vi "CODMn通讯.vi"() -> ()   [LabVIEW 2016, in "斯坦道CODMn新电路板.lvlib"]
uses:
  <vilib>/NI/Modbus Library/API/Wrapper/Create TCP Slave.vi
  <vilib>/Utility/config.llb/Write Key (String).vi
  <vilib>/Plasmionique/MB Master/MB_Master/MB_Master.lvclass
  <vilib>/NI/Modbus Library/API/slave/Modbus Slave.lvclass
  <vilib>/Utility/config.llb/NI_LVConfig.lvlib
  <vilib>/Plasmionique/MB Master/MB Master.lvlib
  <vilib>/NI/Modbus Library/API/Wrapper/API Main.lvlib
panel:
  out "控制命令 2":u16[](array[numeric]) format="%xH"
  out "状态告警区":T1 {"工作状态" items=["空闲"=0, "水样测试"=1, "标样核查"=2, "零点核查"=3, "跨度核查"=4, "空白测试"=5, "平行样测试"=6, "加标回收"=7, "空白校准"=8, "标样校准"=9, "初始化（清洗）"=10, "调试"=22, "填充管路"=30, "清洗管路"=31, "清洗反应杯"=32]; "告警代码" items=["无告警", "缺试剂告警", "缺水样告警", "缺蒸馏水告警", "缺标液告警", "仪表漏液告警", "标定异常告警", "超量程告警", "加热异常", "低试剂预警", "超上限告警", "超下限告警", "仪表内部其他异常", "滴定异常告警", "电极异常告警", "量程切换告警", "参数设置告警", "PH电极电位异常", "电导率电极异常", "浊度光度异常", "溶解氧电极异常", "溶解氧光强异常", "温度异常告警", "PH异常告警", "溶解氧异常告警", "电导率异常告警", "浊度异常告警", "叶绿素异常告警", "藻密度异常告警", "蓝绿藻异常告警", "ORP异常告警", "氨氮异常告警", "清洁刷异常告警", "SD卡异常告警", "蓝牙异常告警", "Wifi异常告警", "流程异常告警"]; "故障代码" items=["无故障", "电机故障", "温度故障", "通讯故障", "滴定故障"]}
  out "测量数据区":T2 {"单位" items=["ug/L", "mg/L", "ppm", "mg/m3", "cm", "ppb", "ug/m3", "%", "nmol/mol", "umol/mol", "MPN/L", "MPN/100ml", "ng/m3", "NTU", "无量纲", "ms/cm", "us/cm", "℃", "mV", "万个/L"]}
  out "状态告警区":u16[](array[numeric])
  out "测量数据区":u16[](array[numeric])
  out "序列号":string
  out "status":bool
  out "关键参数区":T3
  in  "读关键参数区":bool
  in  "读状态告警区":bool
  in  "读测量数据区":bool
  in  "站号":u16(ring) items=["CODMn"=21, "氨氮"=3]
  in  "停止":bool
  in  "启动":bool
  in  "控制命令":u16(ring) items=["启动测量"=1, "标样核查"=2, "零点核查"=3, "跨度核查"=4, "空白测试"=5, "平行样测试"=6, "加标回收"=7, "空白校准"=8, "标样校准"=9, "初始化（清洗）"=10, "停止测试"=11, "仪器重启"=12, "校时"=13, "模式设置"=14, "测量间隔设置"=15]
  in  "控制命令参数":u16[](array[numeric]) format="%04xH"
  in  "VISA Resource":refnum<visa-resource-name>
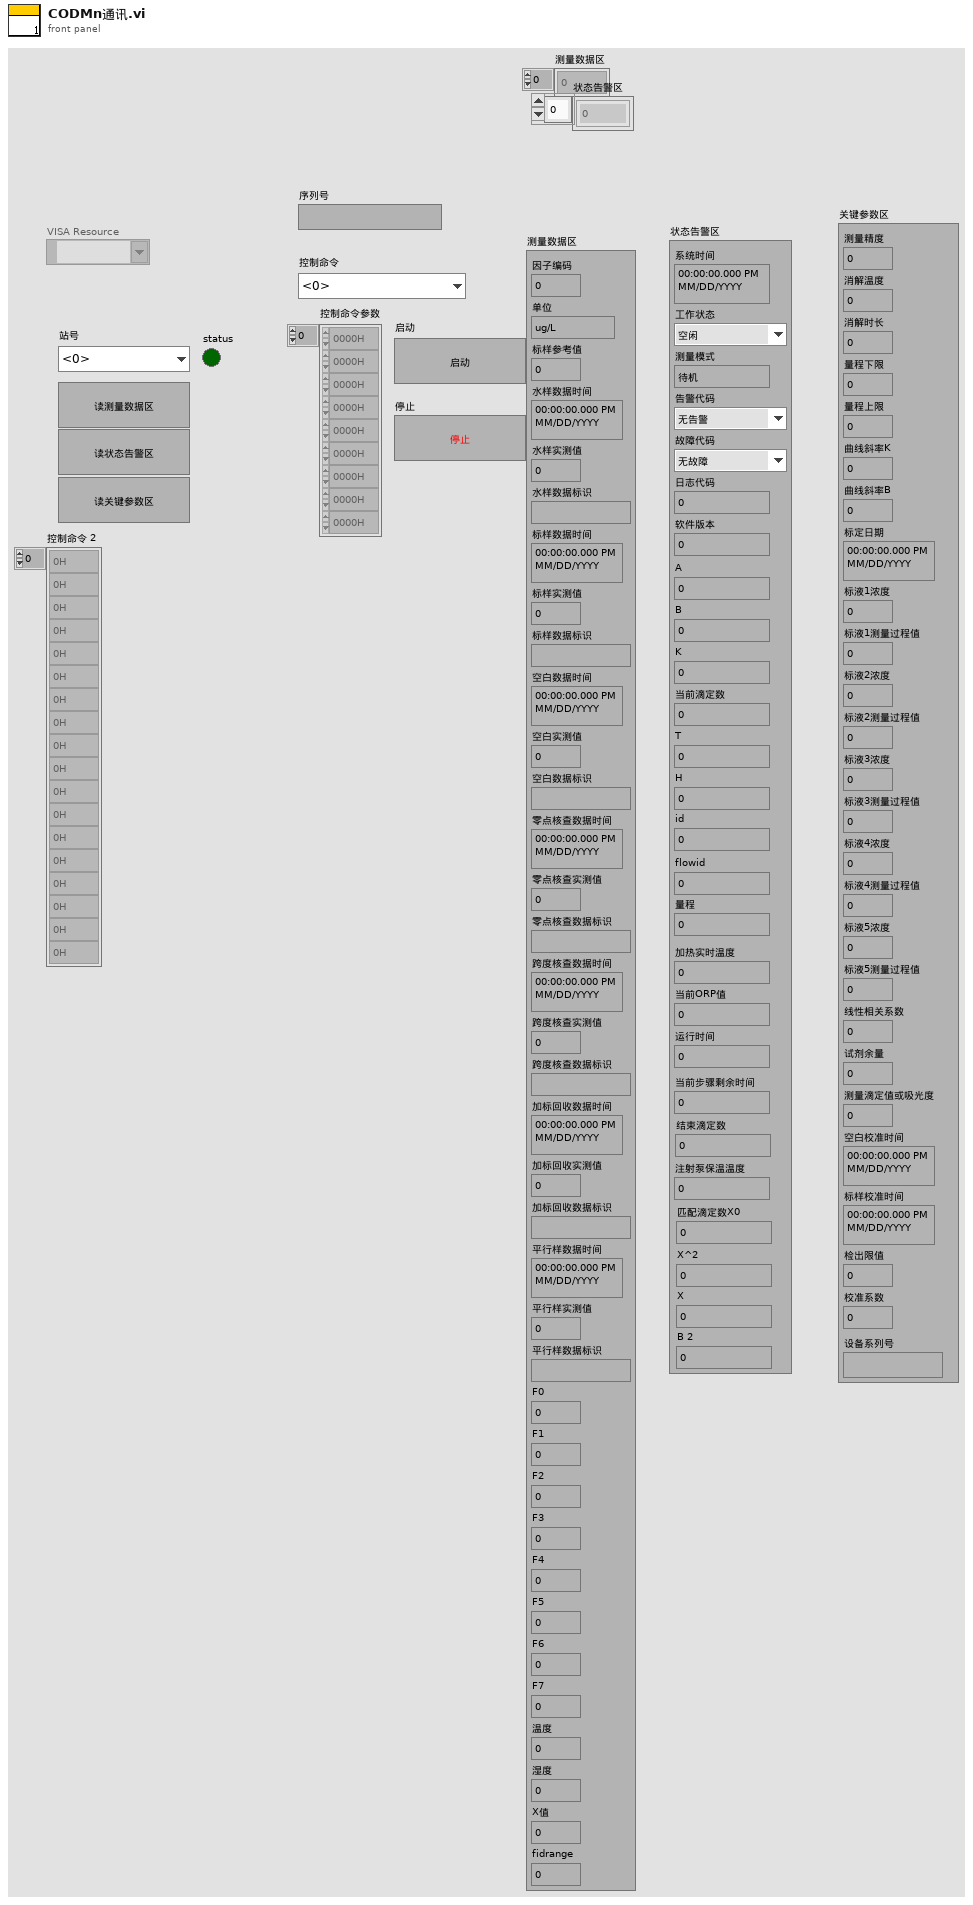
[diagram p1: front panel]
types:
  T1 = cluster{"系统时间":timestamp, "工作状态":u16, "测量模式":enum16{"待机", "连续模式", "周期模式", "定点模式", "受控模式", "手动模式"}, "告警代码":u16, "故障代码":u16, "日志代码":u16, "软件版本":u16, "A":sgl, "B":sgl, "K":sgl, "当前滴定数":sgl, "T":sgl, "H":sgl, "id":u16, "flowid":u16, "量程":u16, "加热实时温度":sgl, "当前ORP值":sgl, "运行时间":sgl, "当前步骤剩余时间":sgl, "结束滴定数":sgl, "注射泵保温温度":sgl, "匹配滴定数X0":u16, "X^2":sgl, "X":sgl, "B 2":sgl}
  T2 = cluster{"因子编码":u32, "单位":u16, "标样参考值":sgl, "水样数据时间":timestamp, "水样实测值":sgl, "水样数据标识":string, "标样数据时间":timestamp, "标样实测值":sgl, "标样数据标识":string, "空白数据时间":timestamp, "空白实测值":sgl, "空白数据标识":string, "零点核查数据时间":timestamp, "零点核查实测值":sgl, "零点核查数据标识":string, "跨度核查数据时间":timestamp, "跨度核查实测值":sgl, "跨度核查数据标识":string, "加标回收数据时间":timestamp, "加标回收实测值":sgl, "加标回收数据标识":string, "平行样数据时间":timestamp, "平行样实测值":sgl, "平行样数据标识":string, "F0":sgl, "F1":sgl, "F2":sgl, "F3":sgl, "F4":sgl, "F5":sgl, "F6":sgl, "F7":sgl, "温度":sgl, "湿度":sgl, "X值":sgl, "fidrange":sgl}
  T3 = cluster{"测量精度":u16, "消解温度":u16, "消解时长":u16, "量程下限":sgl, "量程上限":sgl, "曲线斜率K":sgl, "曲线斜率B":sgl, "标定日期":timestamp, "标液1浓度":sgl, "标液1测量过程值":sgl, "标液2浓度":sgl, "标液2测量过程值":sgl, "标液3浓度":sgl, "标液3测量过程值":sgl, "标液4浓度":sgl, "标液4测量过程值":sgl, "标液5浓度":sgl, "标液5测量过程值":sgl, "线性相关系数":sgl, "试剂余量":u32, "测量滴定值或吸光度":sgl, "空白校准时间":timestamp, "标样校准时间":timestamp, "检出限值":sgl, "校准系数":sgl, "设备系列号":string}
  T4 = typedef "CODMn交互.ctl" = cluster{"COD浓度（mg/L)":dbl, "水样启动时间":timestamp, "加标回收启动时间":timestamp, "CODMn工作状态":enum16{"空闲", "水样测试", "标样核查", "零点核查", "跨度核查", "空白测试", "平行样测试", "加标回收", "空白校准", "标样校准", "初始化（清洗）"}, "多列列表框":i32, "平台试剂余量百分比":sgl, "CODMn仪器参数":cluster{"测量量程":dbl, "测量精度":dbl, "测量间隔":dbl, "消解温度":dbl, "消解时长":dbl, "空白校准时间":timestamp, "曲线截距":dbl, "曲线斜率":dbl, "测量检出限":dbl, "测量信号值":dbl, "线性相关系数":dbl, "二次多项式系数":dbl, "标样校准时间":timestamp, "稀释倍数":dbl, "三项式系数":dbl, "空白标定系数":dbl, "量程系数":dbl, "F0/ORPA":dbl, "F1/ORPB":dbl, "F2/ORPK":dbl, "F3":dbl, "F4":dbl, "F5":dbl, "F6":dbl, "F7":dbl, "X0/滴定数":dbl, "量程":dbl}}
  T5 = cluster{"测量模式":enum16{"水样测量", "标样核查", "零点核查", "跨度核查", "空白测试", "加标回收", "平行样", "校零", "校标"}}
  T6 = typedef "量程选择控件.ctl" = enum32{"L", "H", "AUTO"}
  T7 = cluster{"水样测试量程模式":T6, "标样核查量程模式":T6, "零点核查量程模式":T6, "跨度核查量程模式":T6, "空白测试量程模式":T6, "平行样测试量程模式":T6, "加标回收量程模式":T6, "空白校准量程模式":T6, "标样校准量程模式":T6}
  T8 = cluster{"测量量程":dbl, "测量精度":dbl, "测量间隔":dbl, "消解温度":dbl, "消解时长":dbl, "空白校准时间":timestamp, "曲线截距":dbl, "曲线斜率":dbl, "测量检出限":dbl, "测量信号值":dbl, "线性相关系数":dbl, "二次多项式系数":dbl, "标样校准时间":timestamp, "稀释倍数":dbl, "三项式系数":dbl, "空白标定系数":dbl, "量程系数":dbl, "F0/ORPA":dbl, "F1/ORPB":dbl, "F2/ORPK":dbl, "F3":dbl, "F4":dbl, "F5":dbl, "F6":dbl, "F7":dbl, "X0/滴定数":dbl, "量程":dbl}
  T9 = typedef "NI_LVConfig.lvlib/Config Data RefNum.ctl" = refnum<k1>
  T10 = cluster{"站号":u16, "量程切换":enum32{"H", "L", "AUTO"}, "控制命令":u16, "模式设置":enum16{"待机", "连续模式", "周期模式", "定点模式", "受控模式", "手动模式"}, "测量间隔":u16}
  T11 = enum16{"水样测量", "标样核查", "零点核查", "跨度核查", "空白测试", "加标回收", "平行样", "校零", "校标"}
  T12 = enum8{"Enabled", "Disabled", "Disabled and Grayed Out"}
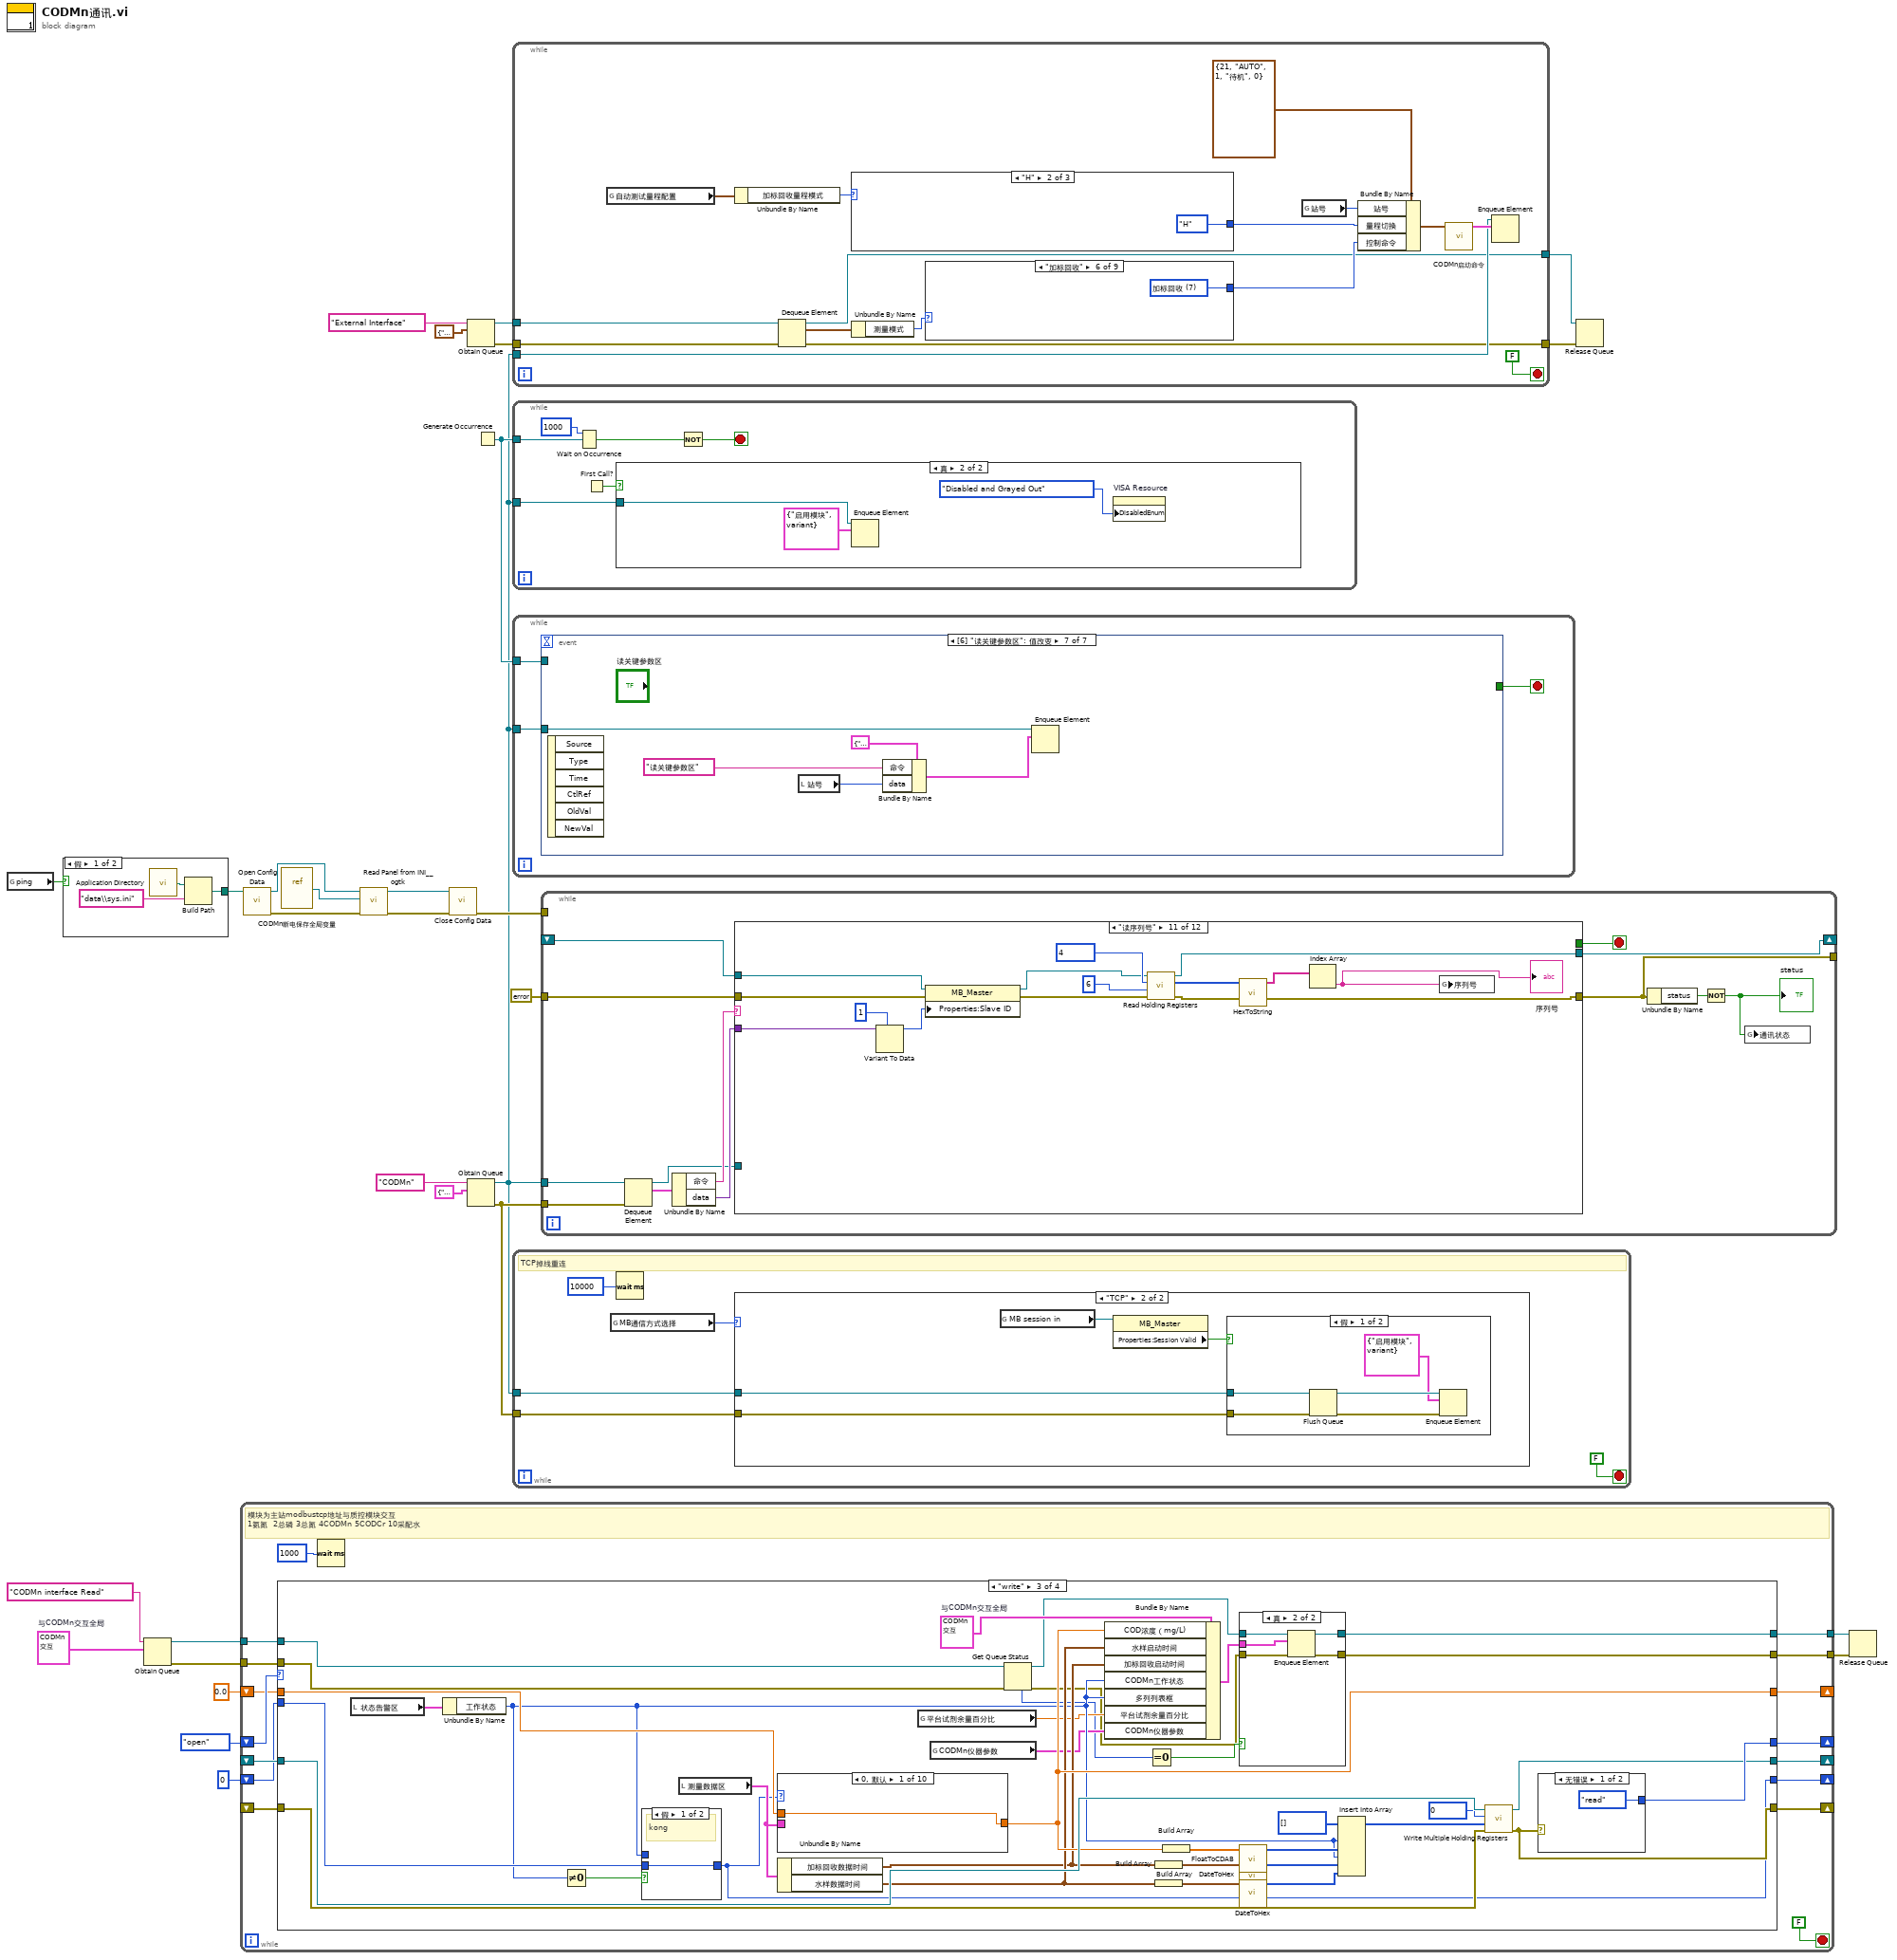
[diagram p0: block diagram]
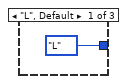
[diagram p2: hidden frame]
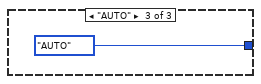
[diagram p3: hidden frame]
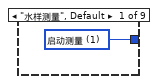
[diagram p4: hidden frame]
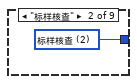
[diagram p5: hidden frame]
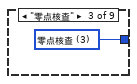
[diagram p6: hidden frame]
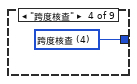
[diagram p7: hidden frame]
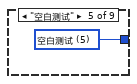
[diagram p8: hidden frame]
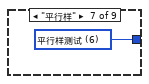
[diagram p9: hidden frame]
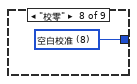
[diagram p10: hidden frame]
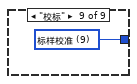
[diagram p11: hidden frame]
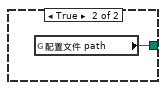
[diagram p12: hidden frame]
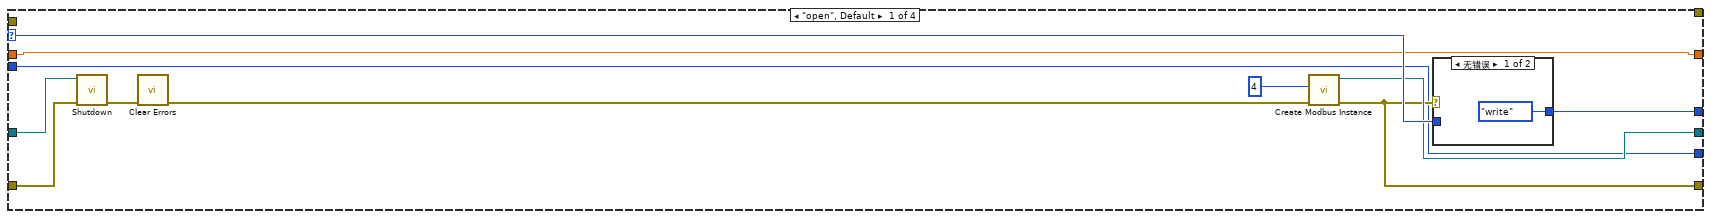
[diagram p15: hidden frame]
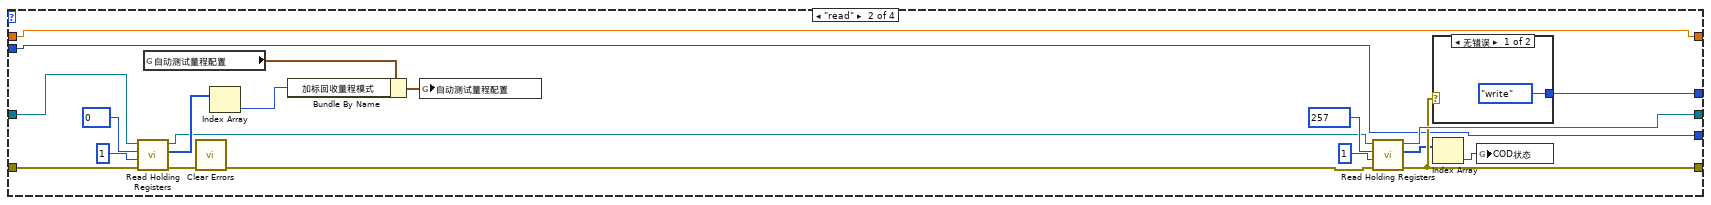
[diagram p17: hidden frame]
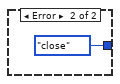
[diagram p18: hidden frame]
diagram:
  w4 = T4 {"COD浓度（mg/L)"=0.0, "水样启动时间"=timestamp(0 s since 1904-01-01), "加标回收启动时间"=timestamp(0 s since 1904-01-01), "CODMn工作状态"=enum."空闲", "多列列表框"=0, "平台试剂余量百分比"=0.0, "CODMn仪器参数"={"测量量程"=0.0, "测量精度"=0.0, "测量间隔"=0.0, "消解温度"=0.0, "消解时长"=0.0, "空白校准时间"=timestamp(0 s since 1904-01-01), "曲线截距"=0.0, "曲线斜率"=0.0, "测量检出限"=0.0, "测量信号值"=0.0, "线性相关系数"=0.0, "二次多项式系数"=0.0, "标样校准时间"=timestamp(0 s since 1904-01-01), "稀释倍数"=0.0, "三项式系数"=0.0, "空白标定系数"=0.0, "量程系数"=0.0, "F0/ORPA"=0.0, "F1/ORPB"=0.0, "F2/ORPK"=0.0, "F3"=0.0, "F4"=0.0, "F5"=0.0, "F6"=0.0, "F7"=0.0, "X0/滴定数"=0.0, "量程"=0.0}}  # 与CODMn交互全局
  n1 = global read "VARCODMn全局变量.vi" "ping"() -> (w17:bool)
  n2 = case shown="假" w17 {
    tunnel: [w30 w33] -> w16
    frame False {
      n3 = call <vilib>:"Application Directory.vi"() -> ("Application Directory"=w32:path)
      n4 = Build Path(base path=w32, name or relative path="data\\sys.ini" ("名称或相对路径")) -> (appended path=w30:path)
    }
    frame True {
      n5 = global read "VARCODMn全局变量.vi" "配置文件 path"() -> (w33:path)
    }
  }
  n6 = Obtain Queue(name (unnamed)="CODMn interface Read" ("写入方名称"), element data type=w4) -> (queue out=w6:refnum<queue>, error out=w1:errorcluster)  [unwired: 3 in, 1 out]
  n7 = while {
    shift-right: [w47] -> _
    shift-left: _ -> [w49]
    shift-right: [w46] -> _
    shift-left: _ -> [w48]
    shift-right: [w43] -> _
    shift-left: enum16{"open", "read", "write", "close"}."open" -> [w44]
    shift-right: [w41] -> _
    shift-left: sgl 0.0 ("标样实测值") -> [w40]
    shift-right: [w39] -> _
    shift-left: u16 0 ("工作状态") -> [w38]
    tunnel: w6 -> [w37]
    tunnel: [w36] -> w3
    tunnel: [w35] -> w2
    tunnel: w1 -> [w34]
    stop <- FALSE stop-if-true
    # "模块为主站modbustcp地址与质控模块交互\n1氨氮  2总磷 3总氮 4CODMn 5CODCr 10采配水"
    n8 = case shown="\"write\"" w44 {
      selector: w44 -> [w60 _ _ _]
      tunnel: w49 -> [w54 w70 w119 w155]
      tunnel: w48 -> [w53 w69 w118 w154]
      tunnel: [w57 w81 w116 w155] -> w47
      tunnel: [w56 w80 w115 w157] -> w46
      tunnel: [w59 w82 w120 enum16{"open", "read", "write", "close"}."open"] -> w43
      tunnel: [w51 w75 w99 w152] -> w41
      tunnel: w40 -> [w51 w75 w112 w152]
      tunnel: [w50 w74 w103 w151] -> w39
      tunnel: w38 -> [w50 w74 w102 w151]
      tunnel: w37 -> [_ _ w93 _]
      tunnel: [_ _ w91 _] -> w36
      tunnel: [_ _ w90 _] -> w35
      tunnel: w34 -> [_ _ w86 _]
      frame "open", Default {
        n9 = call-dynamic "Shutdown.vi"("error in"=w53, "Modbus slave in"=w54) -> ("error out"=w52:errorcluster)  [unwired: 9 in]
        n10 = call <vilib>:"Clear Errors.vi"("error in (no error)"=w52) -> ("error out"=w55:errorcluster)  [unwired: 5 in, 1 out]
        n11 = call-poly <vilib>:"Create Modbus Instance.vi"("error in"=w55, "port (502)"=u16 4) -> ("error out"=w56:errorcluster, "TCP slave instance"=w57:refnum<class "Modbus Slave.lvclass">)  [unwired: 8 in]
        n12 = case shown="无错误" w56 {
          tunnel: w60 -> [_ w62]
          tunnel: [enum16{"open", "read", "write", "close"}."write" w62] -> w59
          frame No Error {
          }
          frame Error {
          }
        }
      }
      frame "read" {
        n13 = call-dynamic <vilib>:"Read Holding Registers.vi"("error in"=w69, "number of inputs"=u16 1, "starting address"=u16 0, "Modbus slave in"=w70) -> ("error out"=w68:errorcluster, "register values"=w73:u16[], "Modbus slave out"=w67:refnum<class "Modbus Slave.lvclass">)  [unwired: 5 in]
        n14 = global read "CODMn断电保存全局变量.vi" "自动测试量程配置"() -> (w65:T7)
        n15 = call <vilib>:"Clear Errors.vi"("error in (no error)"=w68) -> ("error out"=w63:errorcluster)  [unwired: 5 in, 1 out]
        n16 = Index Array(array=w73) -> (element=w64:u16)  [unwired: 1 in]
        n17 = Bundle By Name(cluster=w65, "加标回收量程模式"=w64) -> (w66:T7)
        n18 = global write "CODMn断电保存全局变量.vi" "自动测试量程配置"(w66) -> ()
        n19 = call-dynamic <vilib>:"Read Holding Registers.vi"("error in"=w63, "number of inputs"=u16 1, "starting address"=u16 257, "Modbus slave in"=w67) -> ("error out"=w80:errorcluster, "register values"=w77:u16[], "Modbus slave out"=w81:refnum<class "Modbus Slave.lvclass">)  [unwired: 5 in]
        n20 = case shown="无错误" w80 {
          tunnel: [enum16{"open", "read", "write", "close"}."write" enum16{"open", "read", "write", "close"}."close"] -> w82
          frame No Error {
          }
          frame Error {
          }
        }
        n21 = Index Array(array=w77) -> (element=w76:u16)  [unwired: 1 in]
        n22 = global write "VARCODMn全局变量.vi" "COD状态"(w76) -> ()
      }
      frame "write" {
        w100 = T4 {"COD浓度（mg/L)"=0.0, "水样启动时间"=timestamp(0 s since 1904-01-01), "加标回收启动时间"=timestamp(0 s since 1904-01-01), "CODMn工作状态"=enum."空闲", "多列列表框"=0, "平台试剂余量百分比"=0.0, "CODMn仪器参数"={"测量量程"=0.0, "测量精度"=0.0, "测量间隔"=0.0, "消解温度"=0.0, "消解时长"=0.0, "空白校准时间"=timestamp(0 s since 1904-01-01), "曲线截距"=0.0, "曲线斜率"=0.0, "测量检出限"=0.0, "测量信号值"=0.0, "线性相关系数"=0.0, "二次多项式系数"=0.0, "标样校准时间"=timestamp(0 s since 1904-01-01), "稀释倍数"=0.0, "三项式系数"=0.0, "空白标定系数"=0.0, "量程系数"=0.0, "F0/ORPA"=0.0, "F1/ORPB"=0.0, "F2/ORPK"=0.0, "F3"=0.0, "F4"=0.0, "F5"=0.0, "F6"=0.0, "F7"=0.0, "X0/滴定数"=0.0, "量程"=0.0}}  # 与CODMn交互全局
        n23 = local read "状态告警区"() -> (w101:T1)
        n24 = Unbundle By Name(w101) -> ("工作状态"=w96:u16)
        n25 = Not Equal To 0?(x=w96) -> (x != 0?=w104:bool)
        n26 = case shown="假" w104 {
          tunnel: w96 -> [_ w129]
          tunnel: [w128 w129] -> w103
          tunnel: w102 -> [w128 _]
          frame False {
            # "kong"
          }
          frame True {
            # "..."
          }
        }
        n27 = local read "测量数据区"() -> (w109:T2)
        n28 = case shown="0, 默认" w103 {
          tunnel: [w130 w132 w134 w136 w138 w140 w142 w144 w146 w148] -> w99
          tunnel: w112 -> [w130 _ _ _ _ _ _ _ _ _]
          tunnel: w109 -> [_ w131 w133 w135 w137 w139 w141 w143 w145 w147]
          frame 0, Default {
          }
          frame 1 {
            n29 = Unbundle By Name(w131) -> ("水样实测值"=w132:sgl)
          }
          frame 2 {
            n30 = Unbundle By Name(w133) -> ("标样实测值"=w134:sgl)
          }
          frame 3 {
            n31 = Unbundle By Name(w135) -> ("零点核查实测值"=w136:sgl)
          }
          frame 4 {
            n32 = Unbundle By Name(w137) -> ("跨度核查实测值"=w138:sgl)
          }
          frame 5 {
            n33 = Unbundle By Name(w139) -> ("空白实测值"=w140:sgl)
          }
          frame 6 {
            n34 = Unbundle By Name(w141) -> ("平行样实测值"=w142:sgl)
          }
          frame 7 {
            n35 = Unbundle By Name(w143) -> ("加标回收实测值"=w144:sgl)
          }
          frame 8 {
            n36 = Unbundle By Name(w145) -> ("空白实测值"=w146:sgl)
          }
          frame 9 {
            n37 = Unbundle By Name(w147) -> ("标样实测值"=w148:sgl)
          }
        }
        n38 = Unbundle By Name(w109) -> ("加标回收数据时间"=w97:timestamp, "水样数据时间"=w98:timestamp)
        n39 = global read "VARCODMn全局变量.vi" "平台试剂余量百分比"() -> (w95:sgl)
        n40 = global read "CODMn断电保存全局变量.vi" "CODMn仪器参数"() -> (w94:T8)
        n41 = Get Queue Status(queue=w93, error in (no error)=w86) -> (queue out=w89:refnum<queue>, error out=w85:errorcluster, # elements in queue=w88:i32)  [unwired: 1 in, 5 out]
        n42 = Bundle By Name(cluster=w100, "COD浓度（mg/L)"=w99, "水样启动时间"=w98, "加标回收启动时间"=w97, "CODMn工作状态"=w96, "多列列表框"=w96, "平台试剂余量百分比"=w95, "CODMn仪器参数"=w94) -> (w92:T4)
        n43 = Equal To 0?(x=w88) -> (x = 0?=w87:bool)
        n44 = Build Array(w97) -> (w108:timestamp[])
        n45 = Build Array(w98) -> (w106:timestamp[])
        n46 = Build Array(w99) -> (w111:sgl[])
        n47 = case shown="真" w87 {
          tunnel: w89 -> [w122 w127]
          tunnel: w92 -> [_ w126]
          tunnel: [w122 w125] -> w91
          tunnel: [w121 w124] -> w90
          tunnel: w85 -> [w121 w123]
          frame False {
          }
          frame True {
            n48 = Enqueue Element(queue=w127, element=w126, error in (no error)=w123) -> (queue out=w125:refnum<queue>, error out=w124:errorcluster)  [unwired: 1 in, 1 out]
          }
        }
        n49 = call "FloatToCDAB.vi"("浮点数"=w111) -> ("CDAB整形输出"=w110:u16[])  [unwired: 10 in]
        n50 = call "DateToHex.vi"("DATE"=w108) -> ("数组"=w107:u16[])  [unwired: 10 in]
        n51 = call "DateToHex.vi"("DATE"=w106) -> ("数组"=w105:u16[])  [unwired: 10 in]
        n52 = Insert Into Array(array=u16[] [] ("values"), new element #1=w96, new element #2=w110, new element #3=w96, new element #4=w107, new element #5=w105) -> (w113:u16[])  [unwired: 1 in]
        n53 = call-dynamic "Write Multiple Holding Registers.vi"("error in"=w118, "registers to write"=w113, "starting address"=u16 0, "Modbus slave in"=w119) -> ("error out"=w115:errorcluster, "Modbus slave out"=w116:refnum<class "Modbus Slave.lvclass">)  [unwired: 6 in]
        n54 = case shown="无错误" w115 {
          tunnel: [enum16{"open", "read", "write", "close"}."read" enum16{"open", "read", "write", "close"}."close"] -> w120
          frame No Error {
          }
          frame Error {
          }
        }
      }
      frame "close" {
        n55 = call-dynamic "Shutdown.vi"("error in"=w154, "Modbus slave in"=w155) -> ("error out"=w153:errorcluster)  [unwired: 9 in]
        n56 = call <vilib>:"Clear Errors.vi"("error in (no error)"=w153) -> ("error out"=w157:errorcluster)  [unwired: 5 in, 1 out]
      }
    }
    n57 = Wait (ms)(milliseconds to wait=u32 1000 ("等待时间（毫秒）")) -> ()  [unwired: 1 out]
  }
  n58 = call <vilib>:"Open Config Data.vi"("configuration file path"=w16) -> ("error out"=w24:errorcluster, "refnum"=w21:T9)  [unwired: 8 in, 1 out]
  n59 = vi-ref "CODMn断电保存全局变量.vi"() -> (w22:refnum<vi>)
  n60 = call <userlib>:"Read Panel from INI__ogtk.vi"("error in (no error)"=w24, "VI ref"=w22, "refnum"=w21) -> ("error out"=w25:errorcluster, "refnum out"=w23:T9)  [unwired: 7 in]
  n61 = call <vilib>:"Close Config Data.vi"("error in (no error)"=w25, "refnum"=w23) -> ("error out"=w20:errorcluster)  [unwired: 8 in, 1 out]
  n62 = Obtain Queue(name (unnamed)="External Interface" ("名称（未命名）"), element data type=T5 {"测量模式"=enum."水样测量"} ("元素")) -> (queue out=w13:refnum<queue>, error out=w12:errorcluster)  [unwired: 3 in, 1 out]
  n63 = Obtain Queue(name (unnamed)="CODMn" ("名称（未命名）"), element data type=cluster{"命令":string, "data":variant} {"命令"="", "data"=variant}) -> (queue out=w11:refnum<queue>, error out=w18:errorcluster)  [unwired: 3 in, 1 out]
  n64 = Generate Occurrence() -> (w26:refnum<k4>)
  n65 = while {
    tunnel: w13 -> [w173]
    tunnel: w12 -> [w172]
    tunnel: w11 -> [w164]
    tunnel: [w163] -> w10
    tunnel: [w162] -> w9
    stop <- FALSE stop-if-true
    n66 = global read "CODMn断电保存全局变量.vi" "自动测试量程配置"() -> (w160:T7)
    n67 = Unbundle By Name(w160) -> ("加标回收量程模式"=w159:T6)
    n68 = Dequeue Element(queue=w173, error in (no error)=w172) -> (queue out=w163:refnum<queue>, element=w167:T5, error out=w162:errorcluster)  [unwired: 1 in, 1 out]
    n69 = case shown="\"H\"" w159 {
      tunnel: [enum32{"H", "L", "AUTO"}."L" ("量程切换") enum32{"H", "L", "AUTO"}."H" ("量程切换") enum32{"H", "L", "AUTO"}."AUTO" ("量程切换")] -> w158
      frame "L", Default {
      }
      frame "H" {
      }
      frame "AUTO" {
      }
    }
    n70 = Unbundle By Name(w167) -> ("测量模式"=w166:T11)
    n71 = case shown="\"加标回收\"" w166 {
      tunnel: [w177 w178 w179 w180 w181 w182 w183 w184 w185] -> w165
      frame "水样测量", Default {
        w177 = u16 1 items=["启动测量"=1, "标样核查"=2, "零点核查"=3, "跨度核查"=4, "空白测试"=5, "平行样测试"=6, "加标回收"=7, "空白校准"=8, "标样校准"=9, "初始化（清洗）"=10, "停止测试"=11, "仪器重启"=12, "校时"=13, "模式设置"=14, "测量间隔设置"=15, "调试"=22, "填充管路"=30, "清洗管路"=31, "清洗反应杯"=32] ("控制命令")
      }
      frame "标样核查" {
        w178 = u16 2 items=["启动测量"=1, "标样核查"=2, "零点核查"=3, "跨度核查"=4, "空白测试"=5, "平行样测试"=6, "加标回收"=7, "空白校准"=8, "标样校准"=9, "初始化（清洗）"=10, "停止测试"=11, "仪器重启"=12, "校时"=13, "模式设置"=14, "测量间隔设置"=15, "调试"=22, "填充管路"=30, "清洗管路"=31, "清洗反应杯"=32] ("控制命令")
      }
      frame "零点核查" {
        w179 = u16 3 items=["启动测量"=1, "标样核查"=2, "零点核查"=3, "跨度核查"=4, "空白测试"=5, "平行样测试"=6, "加标回收"=7, "空白校准"=8, "标样校准"=9, "初始化（清洗）"=10, "停止测试"=11, "仪器重启"=12, "校时"=13, "模式设置"=14, "测量间隔设置"=15, "调试"=22, "填充管路"=30, "清洗管路"=31, "清洗反应杯"=32] ("控制命令")
      }
      frame "跨度核查" {
        w180 = u16 4 items=["启动测量"=1, "标样核查"=2, "零点核查"=3, "跨度核查"=4, "空白测试"=5, "平行样测试"=6, "加标回收"=7, "空白校准"=8, "标样校准"=9, "初始化（清洗）"=10, "停止测试"=11, "仪器重启"=12, "校时"=13, "模式设置"=14, "测量间隔设置"=15, "调试"=22, "填充管路"=30, "清洗管路"=31, "清洗反应杯"=32] ("控制命令")
      }
      frame "空白测试" {
        w181 = u16 5 items=["启动测量"=1, "标样核查"=2, "零点核查"=3, "跨度核查"=4, "空白测试"=5, "平行样测试"=6, "加标回收"=7, "空白校准"=8, "标样校准"=9, "初始化（清洗）"=10, "停止测试"=11, "仪器重启"=12, "校时"=13, "模式设置"=14, "测量间隔设置"=15, "调试"=22, "填充管路"=30, "清洗管路"=31, "清洗反应杯"=32] ("控制命令")
      }
      frame "加标回收" {
        w182 = u16 7 items=["启动测量"=1, "标样核查"=2, "零点核查"=3, "跨度核查"=4, "空白测试"=5, "平行样测试"=6, "加标回收"=7, "空白校准"=8, "标样校准"=9, "初始化（清洗）"=10, "停止测试"=11, "仪器重启"=12, "校时"=13, "模式设置"=14, "测量间隔设置"=15, "调试"=22, "填充管路"=30, "清洗管路"=31, "清洗反应杯"=32] ("控制命令")
      }
      frame "平行样" {
        w183 = u16 6 items=["启动测量"=1, "标样核查"=2, "零点核查"=3, "跨度核查"=4, "空白测试"=5, "平行样测试"=6, "加标回收"=7, "空白校准"=8, "标样校准"=9, "初始化（清洗）"=10, "停止测试"=11, "仪器重启"=12, "校时"=13, "模式设置"=14, "测量间隔设置"=15, "调试"=22, "填充管路"=30, "清洗管路"=31, "清洗反应杯"=32] ("控制命令")
      }
      frame "校零" {
        w184 = u16 8 items=["启动测量"=1, "标样核查"=2, "零点核查"=3, "跨度核查"=4, "空白测试"=5, "平行样测试"=6, "加标回收"=7, "空白校准"=8, "标样校准"=9, "初始化（清洗）"=10, "停止测试"=11, "仪器重启"=12, "校时"=13, "模式设置"=14, "测量间隔设置"=15, "调试"=22, "填充管路"=30, "清洗管路"=31, "清洗反应杯"=32] ("控制命令")
      }
      frame "校标" {
        w185 = u16 9 items=["启动测量"=1, "标样核查"=2, "零点核查"=3, "跨度核查"=4, "空白测试"=5, "平行样测试"=6, "加标回收"=7, "空白校准"=8, "标样校准"=9, "初始化（清洗）"=10, "停止测试"=11, "仪器重启"=12, "校时"=13, "模式设置"=14, "测量间隔设置"=15, "调试"=22, "填充管路"=30, "清洗管路"=31, "清洗反应杯"=32] ("控制命令")
      }
    }
    n72 = global read "CODMn断电保存全局变量.vi" "站号"() -> (w168:u16)
    n73 = Bundle By Name(cluster=T10 {"站号"=21, "量程切换"=enum."AUTO", "控制命令"=1, "模式设置"=enum."待机", "测量间隔"=0} ("参数"), "站号"=w168, "量程切换"=w158, "控制命令"=w165) -> (w169:T10)
    n74 = call "CODMn启动命令.vi"("参数"=w169) -> ("启动命令"=w171:cluster{"命令":string, "data":variant})  [unwired: 10 in]
    n75 = Enqueue Element(queue=w164, element=w171) -> ()  [unwired: 2 in, 3 out]
  }
  n76 = while {
    tunnel: w26 -> [w191]
    tunnel: w11 -> [w187]
    stop <- w188 stop-if-true
    n77 = Wait on Occurrence(2:w191, 3:1000 ("毫秒超时(-1)")) -> (0:w189:bool)  [unwired: 1 in]
    n78 = First Call?() -> (First Call?: T/F=w186:bool)
    n79 = case shown="真" w186 {
      tunnel: w187 -> [_ w193]
      frame False {
      }
      frame True {
        n80 = Enqueue Element(queue=w193, element=cluster{"命令":string, "data":variant} {"命令"="启用模块", "data"=variant} ("元素")) -> ()  [unwired: 2 in, 3 out]
        n81 = property on="VISA Resource" class="VISAName"("DisabledEnum"=T12."Disabled and Grayed Out" ("禁用")) -> ()  [unwired: 2 in, 2 out]
      }
    }
    n82 = Not(x=w189) -> (.not. x?=w188:bool)
  }
  n83 = while {
    tunnel: w11 -> [w197]
    tunnel: w26 -> [w195]
    stop <- w196 stop-if-true
    n84 = event shown="[6] \"读关键参数区\": 值改变" {
      selector: _ -> [_ _ _ _ _ _ _]
      dyn-events: _ -> [_ _ _ _ _ _ _]
      timeout: _ -> [_ _ _ _ _ _ _]
      tunnel: w197 -> [_ _ w218 w225 w231 w236 w241]
      tunnel: [_ _ _ "停止" _ _ _] -> w196
      tunnel: w195 -> [_ _ _ w222 _ _ _]
      event Timeout {
        n85 = event-data() -> ()  [unwired: 1 in, 3 out]
      }
      event "VISA Resource": Value Change {
        n86 = event-data() -> ()  [unwired: 1 in, 6 out]
        n87 = call <vilib>:"Application Directory.vi"() -> ("Application Directory"=w200:path)
        n88 = Build Path(base path=w200, name or relative path="data\\set.ini" ("名称或相对路径")) -> (appended path=w201:path)
        n89 = call <vilib>:"Open Config Data.vi"("configuration file path"=w201) -> ("error out"=w207:errorcluster, "refnum"=w206:T9)  [unwired: 8 in, 1 out]
        n90 = call-poly <vilib>:"Write Key.vi"("section"="CODMn", "error in (no error)"=w207, "value"="VISA Resource", "key"="串口", "refnum"=w206) -> ("error out"=w203:errorcluster, "refnum out"=w199:T9)  [unwired: 4 in, 1 out]
        n91 = call <vilib>:"Close Config Data.vi"("error in (no error)"=w203, "refnum"=w199) -> ()  [unwired: 8 in, 2 out]
      }
      event "启动": Value Change {
        n92 = event-data() -> ()  [unwired: 1 in, 6 out]
        n93 = case shown="默认" "控制命令" {
          tunnel: "控制命令参数" -> [w220 w221]
          tunnel: [w219 w221] -> w208
          frame Default {
            n94 = call "HexToWord.vi"("数组"=w220) -> ("WORD"=w219:u16[])  [unwired: 10 in]
          }
          frame 13 {
          }
        }
        n95 = Swap Bytes(anything="控制命令") -> (byte swapped=w211:u16)
        n96 = call "控制命令区.vi"("控制命令参数"=w208, "控制命令"=w211) -> ("控制命令"=w214:u16[])  [unwired: 9 in]
        n97 = local read "站号"() -> (w213:u16)
        n98 = Bundle("站号"=w213, "控制命令"=w214) -> (w212:cluster{"站号":u16, "控制命令":u16[]})  [unwired: 1 in]
        n99 = Bundle By Name(cluster=cluster{"命令":string, "data":variant} {"命令"="", "data"=variant} ("元素"), "命令"="启动", "data"=w212) -> (w216:cluster{"命令":string, "data":variant})
        n100 = Enqueue Element(queue=w218, element=w216) -> ()  [unwired: 2 in, 3 out]
      }
      event "停止": Value Change {
        n101 = event-data() -> ()  [unwired: 1 in, 6 out]
        n102 = Set Occurrence(w222) -> ()
        n103 = Flush Queue(queue=w225) -> (queue out=w224:refnum<queue>)  [unwired: 1 in, 2 out]
        n104 = Enqueue Element(queue=w224, element=cluster{"命令":string, "data":variant} {"命令"="shutdown", "data"=variant} ("元素")) -> ()  [unwired: 2 in, 3 out]
      }
      event "读测量数据区": Value Change {
        n105 = event-data() -> ()  [unwired: 1 in, 6 out]
        n106 = Bundle By Name(cluster=cluster{"命令":string, "data":variant} {"命令"="", "data"=variant} ("元素"), "命令"="读测量数据区", "data"="站号") -> (w229:cluster{"命令":string, "data":variant})
        n107 = Enqueue Element(queue=w231, element=w229) -> ()  [unwired: 2 in, 3 out]
      }
      event "读状态告警区": Value Change {
        n108 = event-data() -> ()  [unwired: 1 in, 6 out]
        n109 = local read "站号"() -> (w232:u16)
        n110 = Bundle By Name(cluster=cluster{"命令":string, "data":variant} {"命令"="", "data"=variant} ("元素"), "命令"="读状态告警区", "data"=w232) -> (w234:cluster{"命令":string, "data":variant})
        n111 = Enqueue Element(queue=w236, element=w234) -> ()  [unwired: 2 in, 3 out]
      }
      event "读关键参数区": Value Change {
        n112 = event-data() -> ()  [unwired: 1 in, 6 out]
        n113 = local read "站号"() -> (w237:u16)
        n114 = Bundle By Name(cluster=cluster{"命令":string, "data":variant} {"命令"="", "data"=variant} ("元素"), "命令"="读关键参数区", "data"=w237) -> (w239:cluster{"命令":string, "data":variant})
        n115 = Enqueue Element(queue=w241, element=w239) -> ()  [unwired: 2 in, 3 out]
      }
    }
  }
  n116 = while "While循环" {
    tunnel: w11 -> [w244]
    tunnel: w18 -> [w243]
    stop <- FALSE stop-if-true
    # "TCP掉线重连"
    n117 = global read "CODMn断电保存全局变量.vi" "MB通信方式选择"() -> (w242:enum16{"串口", "TCP"})
    n118 = Wait (ms)(milliseconds to wait=u32 10000 ("等待时间（毫秒）")) -> ()  [unwired: 1 out]
    n119 = case shown="\"TCP\"" w242 {
      tunnel: w244 -> [_ w249]
      tunnel: w243 -> [_ w248]
      frame "串口", Default {
      }
      frame "TCP" {
        n120 = global read "VARCODMn全局变量.vi" "MB session in"() -> (w247:refnum<class "MB_Master.lvclass">)
        n121 = property class="MB_Master"(reference=w247) -> ("Properties:Session Valid"=w250:bool)  [unwired: 1 in, 2 out]
        n122 = case shown="假" w250 {
          tunnel: w249 -> [w253 _]
          tunnel: w248 -> [w252 _]
          frame False {
            n123 = Flush Queue(queue=w253, error in (no error)=w252) -> (queue out=w255:refnum<queue>, error out=w254:errorcluster)  [unwired: 1 out]
            n124 = Enqueue Element(queue=w255, element=cluster{"命令":string, "data":variant} {"命令"="启用模块", "data"=variant} ("元素"), error in (no error)=w254) -> ()  [unwired: 1 in, 3 out]
          }
          frame True {
          }
        }
      }
    }
  }
  n125 = while {
    tunnel: w11 -> [w268]
    tunnel: w18 -> [w267]
    shift-right: [w265] -> _
    shift-left: _ -> [w264]
    tunnel: errorcluster {"status"=FALSE, "code"=0, "source"=""} ("error out") -> [w263]
    tunnel: [w258] -> _
    tunnel: w20 -> [_]
    stop <- w266 stop-if-true
    n126 = Dequeue Element(queue=w268, error in (no error)=w267) -> (queue out=w259:refnum<queue>, element=w261:cluster{"命令":string, "data":variant})  [unwired: 1 in, 2 out]
    n127 = Unbundle By Name(w261) -> ("命令"=w262:string, "data"=w260:variant)
    n128 = case shown="\"读序列号\"" w262 {
      tunnel: w260 -> [_ _ _ w287 w298 w315 w327 w336 w346 w362 w377 _]
      tunnel: w259 -> [_ _ _ _ _ _ _ _ _ _ _ w390]
      tunnel: [_ _ _ _ _ _ _ _ _ _ _ TRUE] -> w266
      tunnel: [w269 w272 w274 w290 w301 w317 w329 w341 w355 w369 w384 w386] -> w265
      tunnel: [w270 w271 w275 w289 w300 w316 w328 w330 w344 w358 w385 w387] -> w258
      tunnel: w264 -> [w269 _ w274 w286 w297 w314 w326 w335 w349 w365 w380 w386]
      tunnel: w263 -> [w270 _ w277 w283 w294 w311 w323 w333 w350 w366 w381 w388]
      frame Default {
      }
      frame "启用模块" {
        n129 = call "MB_api.vi"("STEP"=enum16{"open", "read", "write", "close"}."open") -> ("error out"=w271:errorcluster, "MB session out"=w272:refnum<class "MB_Master.lvclass">)  [unwired: 8 in, 1 out]
        n130 = global write "VARCODMn全局变量.vi" "MB session in"(w272) -> ()
      }
      frame "停用模块" {
        n131 = call-dynamic "Close Session.vi"("error in (no error)"=w277, "MB session in"=w274) -> ("error out"=w276:errorcluster)  [unwired: 9 in]
        n132 = call <vilib>:"Clear Errors.vi"("error in (no error)"=w276) -> ("error out"=w275:errorcluster)  [unwired: 5 in, 1 out]
      }
      frame "启动" {
        n133 = Variant To Data(type=cluster{"站号":u16, "控制命令":u16[]} {"站号"=0, "控制命令"=[]} ("输出簇"), Variant=w287) -> (data=w281:cluster{"站号":u16, "控制命令":u16[]})  [unwired: 1 in, 1 out]
        n134 = Unbundle By Name(w281) -> ("站号"=w280:u16, "控制命令"=w278:u16[])
        n135 = property class="MB_Master"(reference=w286, error in=w283, "Properties:Slave ID"=w280) -> (reference out=w285:refnum<class "MB_Master.lvclass">, error out=w284:errorcluster)
        n136 = Index Array(array=w278) -> (element=w279:u16)  [unwired: 1 in]
        n137 = global write "VARCODMn全局变量.vi" "控制命令"(w279) -> ()
        n138 = call <vilib>:"Write Multiple Registers.vi"("error in (no error)"=w284, "values"=w278, "starting address"=u16 4608, "MB session in"=w285) -> ("error out"=w289:errorcluster, "MB session out"=w290:refnum<class "MB_Master.lvclass">)  [unwired: 6 in]
      }
      frame "盲样测试" {
        n139 = Variant To Data(type=0, Variant=w298) -> (data=w291:i32)  [unwired: 1 in, 1 out]
        n140 = property class="MB_Master"(reference=w297, error in=w294, "Properties:Slave ID"=w291) -> (reference out=w296:refnum<class "MB_Master.lvclass">, error out=w295:errorcluster)
        n141 = case shown="默认" w291 {
          tunnel: [u16[] [] ("values") u16[] [33539, 0] ("values") u16[] [23555, 0] ("values")] -> w293
          frame Default {
          }
          frame 1 {
            # "总磷盲样测试命令"
          }
          frame 3 {
            # "氨氮盲样测试"
          }
        }
        n142 = call <vilib>:"Write Multiple Registers.vi"("error in (no error)"=w295, "values"=w293, "starting address"=u16 24592, "MB session in"=w296) -> ("error out"=w300:errorcluster, "MB session out"=w301:refnum<class "MB_Master.lvclass">)  [unwired: 6 in]
      }
      frame "debug" {
        n143 = Variant To Data(type=cluster{"站号":u16, "控制命令":u16[]} {"站号"=0, "控制命令"=[]} ("输出簇"), Variant=w315) -> (data=w309:cluster{"站号":u16, "控制命令":u16[]})  [unwired: 1 in, 1 out]
        n144 = Unbundle By Name(w309) -> ("站号"=w308:u16, "控制命令"=w306:u16[])
        "控制命令 2" <- w306
        n145 = property class="MB_Master"(reference=w314, error in=w311, "Properties:Slave ID"=w308) -> (reference out=w313:refnum<class "MB_Master.lvclass">, error out=w312:errorcluster)
        n146 = Index Array(array=w306) -> (element=w307:u16)  [unwired: 1 in]
        n147 = global write "VARCODMn全局变量.vi" "控制命令"(w307) -> ()
        n148 = call <vilib>:"Write Multiple Registers.vi"("error in (no error)"=w312, "values"=w306, "starting address"=u16 24594, "MB session in"=w313) -> ("error out"=w316:errorcluster, "MB session out"=w317:refnum<class "MB_Master.lvclass">)  [unwired: 6 in]
      }
      frame "单步控制" {
        n149 = Variant To Data(type=cluster{"站号":u16, "控制命令":u16[]} {"站号"=0, "控制命令"=[]} ("输出簇"), Variant=w327) -> (data=w321:cluster{"站号":u16, "控制命令":u16[]})  [unwired: 1 in, 1 out]
        n150 = Unbundle By Name(w321) -> ("站号"=w320:u16, "控制命令"=w319:u16[])
        n151 = property class="MB_Master"(reference=w326, error in=w323, "Properties:Slave ID"=w320) -> (reference out=w325:refnum<class "MB_Master.lvclass">, error out=w324:errorcluster)
        n152 = call <vilib>:"Write Multiple Registers.vi"("error in (no error)"=w324, "values"=w319, "starting address"=u16 24610, "MB session in"=w325) -> ("error out"=w328:errorcluster, "MB session out"=w329:refnum<class "MB_Master.lvclass">)  [unwired: 6 in]
      }
      frame "读测量数据区" {
        n153 = Variant To Data(type=u8 1 ("Slave ID"), Variant=w336) -> (data=w337:u8)  [unwired: 1 in, 1 out]
        n154 = property class="MB_Master"(reference=w335, error in=w333, "Properties:Slave ID"=w337) -> (reference out=w334:refnum<class "MB_Master.lvclass">, error out=w332:errorcluster)
        n155 = call <vilib>:"Read Holding Registers.vi"("error in (no error)"=w332, "quantity"=u16 105, "starting address"=u16 4096, "MB session in"=w334) -> ("error out"=w330:errorcluster, "Registers"=w331:u16[], "MB session out"=w341:refnum<class "MB_Master.lvclass">)  [unwired: 5 in]
        n156 = case shown="无错误" w330 {
          tunnel: w331 -> [w343 _]
          frame No Error {
            n157 = call "测量数据区.vi"("数组"=w343) -> ("测量数据区"=w342:T2)  [unwired: 10 in]
            "测量数据区" <- w342
            n158 = global write "VARCODMn全局变量.vi" "测量数据区"(w342) -> ()
            "测量数据区" <- w343
          }
          frame Error {
          }
        }
      }
      frame "读状态告警区" {
        n159 = Variant To Data(type=u8 1 ("Slave ID"), Variant=w346) -> (data=w351:u8)  [unwired: 1 in, 1 out]
        n160 = property class="MB_Master"(reference=w349, error in=w350, "Properties:Slave ID"=w351) -> (reference out=w348:refnum<class "MB_Master.lvclass">, error out=w347:errorcluster)
        n161 = call <vilib>:"Read Holding Registers.vi"("error in (no error)"=w347, "quantity"=u16 40, "starting address"=u16 4224, "MB session in"=w348) -> ("error out"=w344:errorcluster, "Registers"=w345:u16[], "MB session out"=w355:refnum<class "MB_Master.lvclass">)  [unwired: 5 in]
        n162 = case shown="无错误" w344 {
          tunnel: w345 -> [w357 _]
          frame No Error {
            n163 = call "状态告警区.vi"("数组"=w357) -> ("状态告警区"=w356:T1)  [unwired: 10 in]
            "状态告警区" <- w356
            n164 = global write "VARCODMn全局变量.vi" "状态告警区"(w356) -> ()
            "状态告警区" <- w357
          }
          frame Error {
          }
        }
      }
      frame "读关键参数区" {
        n165 = Variant To Data(type=u8 1 ("Slave ID"), Variant=w362) -> (data=w360:u8)  [unwired: 1 in, 1 out]
        n166 = property class="MB_Master"(reference=w365, error in=w366, "Properties:Slave ID"=w360) -> (reference out=w364:refnum<class "MB_Master.lvclass">, error out=w363:errorcluster)
        n167 = call <vilib>:"Read Holding Registers.vi"("error in (no error)"=w363, "quantity"=u16 19, "starting address"=u16 4256, "MB session in"=w364) -> ("error out"=w358:errorcluster, "Registers"=w359:u16[], "MB session out"=w369:refnum<class "MB_Master.lvclass">)  [unwired: 5 in]
        n168 = case shown="无错误" w358 {
          tunnel: w359 -> [w371 _]
          frame No Error {
            n169 = call "关键参数区.vi"("数组"=w371) -> ("关键参数区"=w370:T3)  [unwired: 10 in]
            "关键参数区" <- w370
            n170 = global write "VARCODMn全局变量.vi" "关键参数区"(w370) -> ()
          }
          frame Error {
          }
        }
      }
      frame "读序列号" {
        n171 = Variant To Data(type=u8 1 ("Slave ID"), Variant=w377) -> (data=w375:u8)  [unwired: 1 in, 1 out]
        n172 = property class="MB_Master"(reference=w380, error in=w381, "Properties:Slave ID"=w375) -> (reference out=w379:refnum<class "MB_Master.lvclass">, error out=w378:errorcluster)
        n173 = call <vilib>:"Read Holding Registers.vi"("error in (no error)"=w378, "quantity"=u16 6, "starting address"=u16 4, "MB session in"=w379) -> ("error out"=w385:errorcluster, "Registers"=w374:u16[], "MB session out"=w384:refnum<class "MB_Master.lvclass">)  [unwired: 5 in]
        n174 = call "HexToString.vi"("数组"=w374) -> ("STRING"=w373:string[])  [unwired: 10 in]
        n175 = Index Array(array=w373) -> (element=w372:string)  [unwired: 1 in]
        "序列号" <- w372
        n176 = global write "VARCODMn全局变量.vi" "序列号"(w372) -> ()
      }
      frame "shutdown" {
        n177 = call-dynamic "Close Session.vi"("error in (no error)"=w388, "MB session in"=w386) -> ("error out"=w387:errorcluster)  [unwired: 9 in]
        n178 = Flush Queue(queue=w390) -> (queue out=w389:refnum<queue>)  [unwired: 1 in, 2 out]
        n179 = Release Queue(queue=w389) -> ()  [unwired: 2 in, 3 out]
      }
    }
    n180 = Unbundle By Name(w258) -> ("status"=w257:bool)
    n181 = Not(x=w257) -> (.not. x?=w256:bool)
    "status" <- w256
    n182 = global write "VARCODMn全局变量.vi" "通讯状态"(w256) -> ()
  }
  n183 = Release Queue(queue=w10, error in (no error)=w9) -> ()  [unwired: 1 in, 3 out]
  n184 = Release Queue(queue=w3, error in (no error)=w2) -> ()  [unwired: 1 in, 3 out]
